vi "Log_ADAM_scan_table.vi"() -> ()   [LabVIEW 2012]
uses:
  ADAM Client/Sub VIs/ADAM Controls/Channel_State.ctl
  Anemometry/Anemometry Sub Vis/Globals/Constants_global.vi
  Anemometry/Anemometry Sub Vis/Globals/Preference_global.vi
  ADAM_Global.vi
  Anemometry/Anemometry Sub Vis/Globals/Meas_global.vi
panel:
  in  "Averaging time (Seconds)":dbl=60.0
  out "Current time":string
  out "Started Time":string
  in  "stop":bool
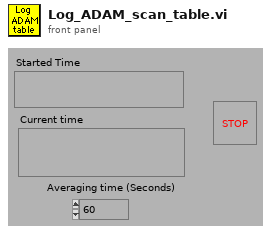
[diagram p1: front panel]
types:
  T1 = enum16{"On", "Off", "Always On", "Always Off", "Delete"}
  T2 = typedef "Channel_State.ctl" = enum16{"On", "Off", "Always On", "Always Off"}
  T3 = enum16{"Load ADAM setup from excel file", "Save ADAM setup to excel file"}
  T4 = cluster{"second":i32, "minute":i32, "hour":i32, "day of month":i32, "month":i32, "year":i32, "day of week":i32, "day of year":i32, "is DST":i32}
  T5 = typedef "Client_State_Cluster.ctl" = cluster{"Client Name":string, "Traverse level State":T6, "People to Email":string[], "Next Contact Time":dbl}
  T6 = typedef "Traverse_Level_State.ctl" = enum16{"Running", "Complete"}
  T7 = typedef "Server_Control.ctl" = cluster{"Channel Name to control":string, "Channel sharing":enum16{"Channel Unshared", "Channel Shared by Rig", "Channel Shared by Group"}, "Default Value":dbl, "Client Array":string[], "Time Stamp":timestamp, "Do Not Reset":bool}
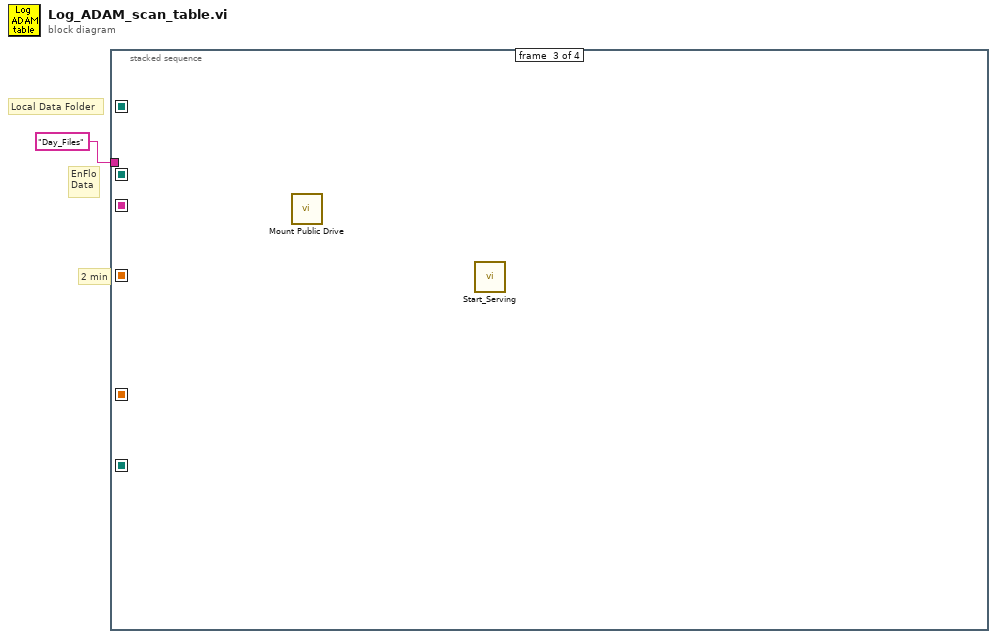
[diagram p0: block diagram]
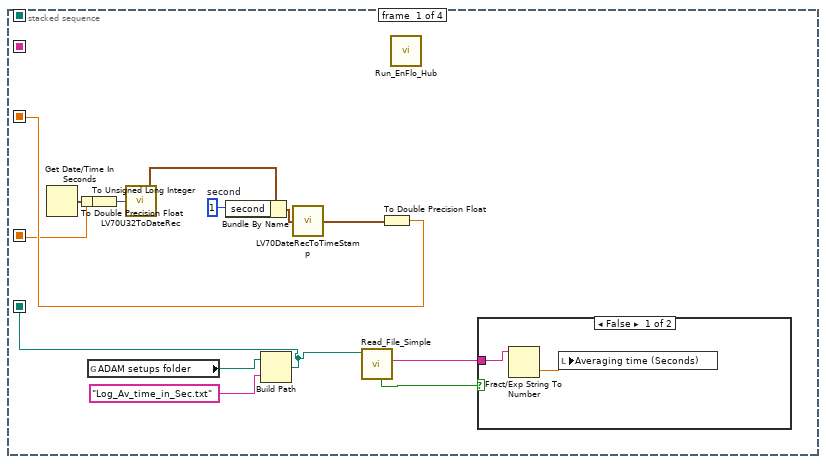
[diagram p2: hidden frame]
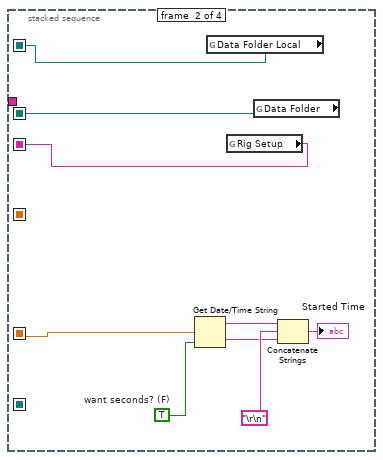
[diagram p4: hidden frame]
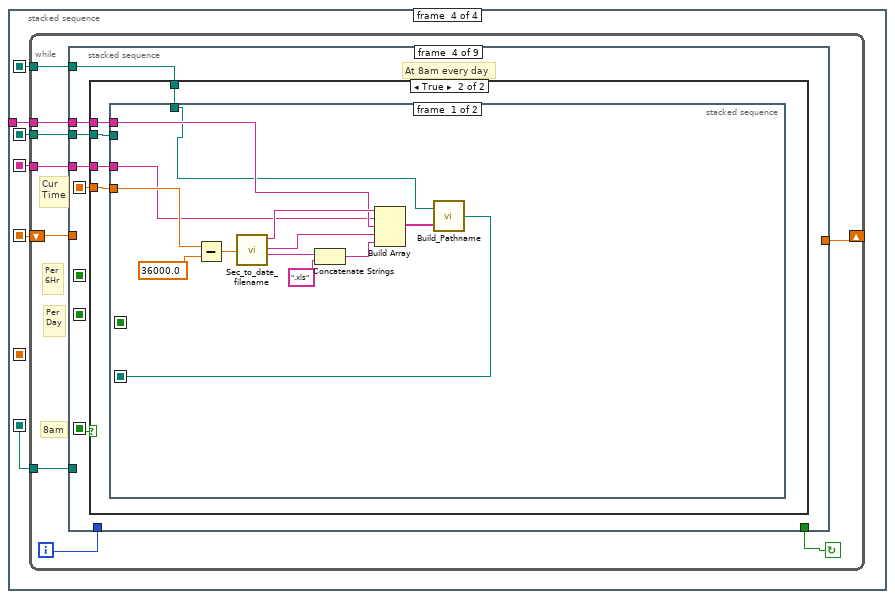
[diagram p5: hidden frame]
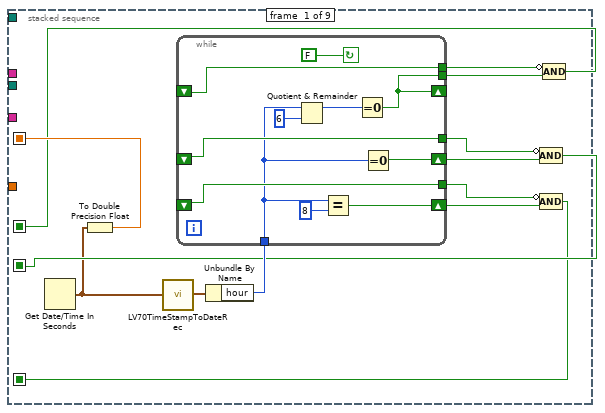
[diagram p6: hidden frame]
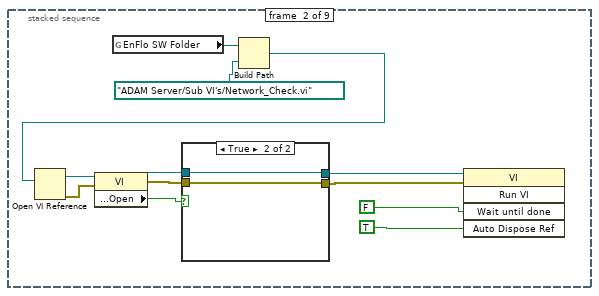
[diagram p7: hidden frame]
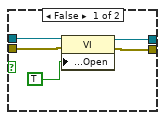
[diagram p8: hidden frame]
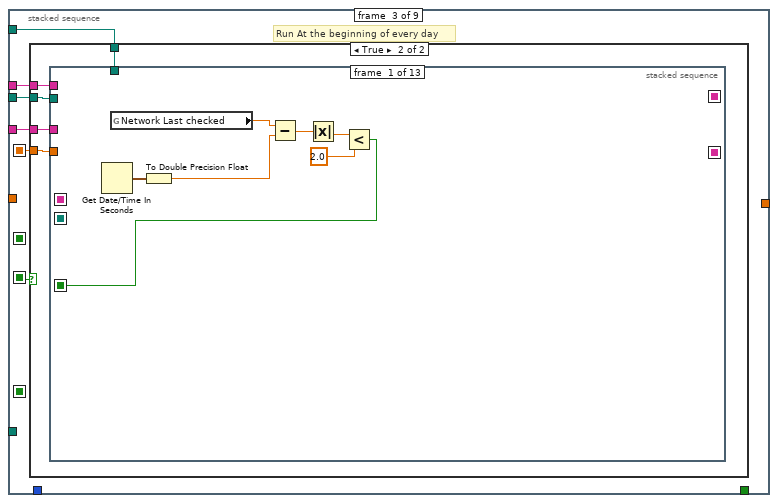
[diagram p9: hidden frame]
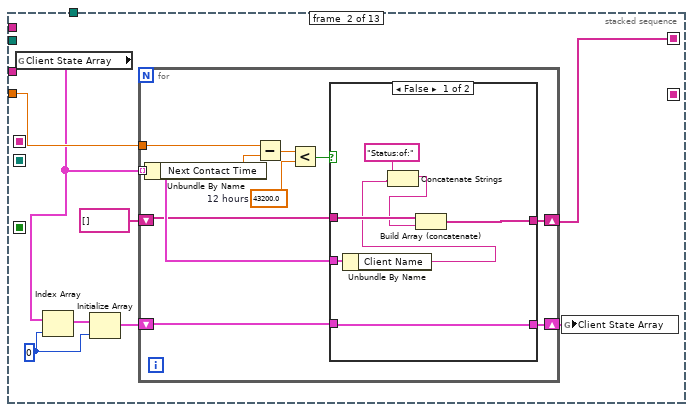
[diagram p11: hidden frame]
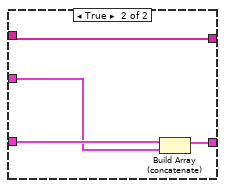
[diagram p12: hidden frame]
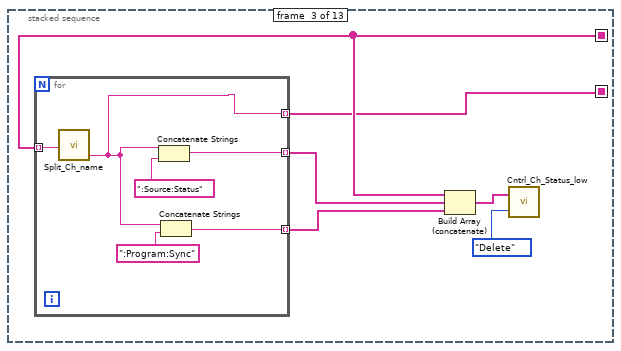
[diagram p13: hidden frame]
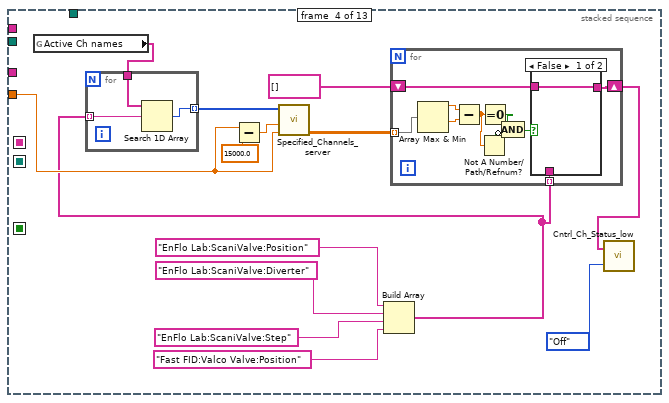
[diagram p14: hidden frame]
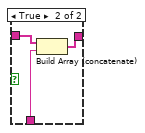
[diagram p15: hidden frame]
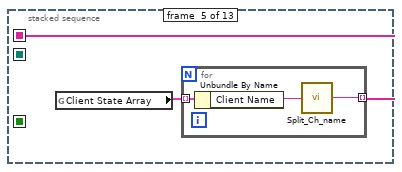
[diagram p16: hidden frame]
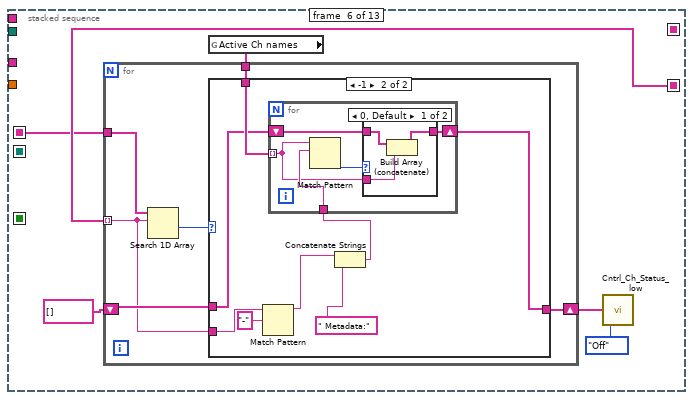
[diagram p17: hidden frame]
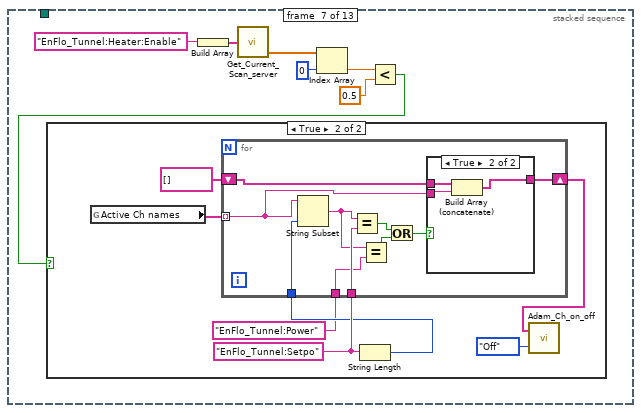
[diagram p20: hidden frame]
diagram:
  # "Local Data Folder"
  # "EnFlo\nData"
  # "2 min"
  n1 = stacked-sequence {
    seq-local: [w12 _ _ _] -> [_ _ _ w31]
    seq-local: [w11 _ _ _] -> [_ w25 _ _]
    seq-local: [_ w19 _ _] -> [_ _ _ w30]
    seq-local: [w4 _ _ _] -> [_ _ _ w28]
    seq-local: [_ w18 _ _] -> [_ _ _ w27]
    seq-local: [_ w17 _ _] -> [_ _ _ w26]
    tunnel: "Day_Files" ("Input Element") -> [_ _ _ w29]
    frame #0 {
      w14 = 1  # second
      n2 = Get Date/Time In Seconds() -> (seconds since 1Jan1904=w8:timestamp)
      n3 = To Double Precision Float(number=w8) -> (double precision float=w11:dbl)
      n4 = global read "Constants_global.vi" "ADAM setups folder"() -> (w6:path)
      n5 = To Unsigned Long Integer(number=w11) -> (unsigned 32bit integer=w10:u32)
      n6 = call <vilib>:"LV70U32ToDateRec.vi"("Time"=w10) -> ("date time rec"=w9:T4)
      n7 = Bundle By Name(cluster=w9, "second"=w14) -> (w13:T4)
      n8 = Build Path(base path=w6, name or relative path="Log_Av_time_in_Sec.txt") -> (appended path=w4:path)
      n9 = call <vilib>:"LV70DateRecToTimeStamp.vi"("date time rec"=w13) -> ("Time Stamp"=w7:timestamp)
      n10 = call "Read_File_Simple.vi"("Filename"=w4) -> ("Error?"=w2:bool, "string"=w3:string)  [unwired: 2 in, 6 out]
      n11 = To Double Precision Float(number=w7) -> (double precision float=w12:dbl)
      n12 = call "Run_EnFlo_Hub.vi"() -> ()  [unwired: 8 out]
      n13 = case shown="False" w2 {
        tunnel: w3 -> [w16 _]
        frame False {
          n14 = Fract/Exp String To Number(string=w16) -> (number=w15:dbl)  [unwired: 4 out]
          n15 = local write "Averaging time (Seconds)"(w15) -> ()
        }
        frame True {
        }
      }
    }
    frame #1 {
      w24 = TRUE  # want seconds? (F)
      n16 = Get Date/Time String(seconds (now)=w25, want seconds? (F)=w24) -> (date string=w22:string, time string=w21:string)  [unwired: 1 out]
      n17 = global read "Constants_global.vi" "Data Folder Local"() -> (w17:path)
      n18 = global read "Preference_global.vi" "Rig Setup"() -> (w18:string)
      n19 = global read "Constants_global.vi" "Data Folder"() -> (w19:path)
      n20 = Concatenate Strings(w22, "\r\n", w21) -> (→"Started Time":string)
    }
    frame #2 {
      n21 = call "Mount Public Drive.vi"() -> ()  [unwired: 12 in]
      n22 = call "Start_Serving.vi"() -> ()  [unwired: 1 out]
    }
    frame #3 {
      n23 = while {
        tunnel: w30 -> [w38]
        shift-left: w31 -> [w40]
        shift-right: [w39] -> _
        tunnel: w29 -> [w35]
        tunnel: w28 -> [w34]
        tunnel: w27 -> [w33]
        tunnel: w26 -> [w32]
        i -> [w37]
        stop <- w36 continue-if-true
        # "8am"
        # "Per\n6Hr"
        # "Per\nDay"
        # "Cur\nTime"
        n24 = stacked-sequence {
          seq-local: [w45 _ _ _ _ _ _ _ _] -> [_ _ w89 _ _ _ _ _ _]
          seq-local: [w52 _ _ _ _ _ _ _ _] -> [_ _ w88 w329 w366 w380 w384 _ _]
          seq-local: [w48 _ _ _ _ _ _ _ _] -> [_ _ _ _ w360 _ _ _ _]
          seq-local: [w41 _ _ _ _ _ _ _ _] -> [_ _ _ w324 _ _ _ _ _]
          tunnel: [_ _ _ _ _ _ w383 _ _] -> w39
          tunnel: w40 -> [_ _ _ _ _ _ w385 _ _]
          tunnel: w38 -> [_ _ w87 w328 _ _ w392 _ _]
          tunnel: w37 -> [_ _ _ _ w359 _ _ _ _]
          tunnel: [_ _ _ _ _ _ _ _ w441] -> w36
          tunnel: w35 -> [_ _ w86 w327 _ _ w393 _ _]
          tunnel: w34 -> [_ _ _ _ _ _ _ _ w440]
          tunnel: w33 -> [_ _ w85 w326 _ _ w386 _ _]
          tunnel: w32 -> [_ _ w84 w325 _ _ w382 _ _]
          frame #0 {
            n25 = Get Date/Time In Seconds() -> (seconds since 1Jan1904=w44:timestamp)
            n26 = To Double Precision Float(number=w44) -> (double precision float=w52:dbl)
            n27 = call <vilib>:"LV70TimeStampToDateRec.vi"("time stamp"=w44) -> ("date time rec"=w53:T4)
            n28 = Unbundle By Name(w53) -> ("hour"=w51:i32)
            n29 = while {
              tunnel: [w59] -> w46
              shift-left: _ -> [w59]
              shift-right: [w60] -> w47
              tunnel: [w61] -> w49
              tunnel: [w62] -> w50
              tunnel: w51 -> [w56]
              shift-left: _ -> [w61]
              shift-right: [w62] -> _
              tunnel: [w57] -> w43
              shift-right: [w54] -> w42
              shift-left: _ -> [w57]
              stop <- FALSE continue-if-true
              n30 = Quotient & Remainder(x=w56, y=6) -> (x-y*floor(x/y)=w63:i32)  [unwired: 1 out]
              n31 = Equal?(x=w56, y=8) -> (x = y?=w54:bool)
              n32 = Equal To 0?(x=w63) -> (x = 0?=w62:bool)
              n33 = Equal To 0?(x=w56) -> (x = 0?=w60:bool)
            }
            n34 = Compound Arithmetic op=AND(invert w46, w47) -> (w45:bool)
            n35 = Compound Arithmetic op=AND(invert w43, w42) -> (w41:bool)
            n36 = Compound Arithmetic op=AND(invert w49, w50) -> (w48:bool)
          }
          frame #1 {
            n37 = global read "Constants_global.vi" "EnFlo SW Folder"() -> (w74:path)
            n38 = Build Path(base path=w74, name or relative path=path "ADAM Server/Sub VI's/Network_Check.vi") -> (appended path=w75:path)
            n39 = Open VI Reference(vi path=w75) -> (vi reference=w71:refnum<vi>, error out=w70:errorcluster)  [unwired: 1 in, 4 out]
            n40 = property class="VI"(reference=w71, error in=w70) -> (reference out=w68:refnum<vi>, error out=w67:errorcluster, "Front Panel Window:Open"=w69:bool)
            n41 = case shown="True" w69 {
              tunnel: w68 -> [w80 w83]
              tunnel: w67 -> [w79 w82]
              tunnel: [w78 w83] -> w66
              tunnel: [w77 w82] -> w65
              frame False {
                n42 = property class="VI"(reference=w80, error in=w79, "Front Panel Window:Open"=TRUE) -> (reference out=w78:refnum<vi>, error out=w77:errorcluster)
              }
              frame True {
              }
            }
            n43 = invoke class="VI" method="Run VI"(reference=w66, error in=w65, "Wait until done"=FALSE, "Auto Dispose Ref"=TRUE) -> ()  [unwired: 1 in, 5 out]
          }
          frame #2 {
            # "Run At the beginning of every day"
            n44 = case shown="True" w89 {
              tunnel: w88 -> [_ w94]
              tunnel: w87 -> [_ w93]
              tunnel: w86 -> [_ w92]
              tunnel: w85 -> [_ w91]
              tunnel: w84 -> [_ w90]
              frame False {
              }
              frame True {
                n45 = stacked-sequence {
                  seq-local: [_ w102 _ _ _ _ _ _ _ _ _ _ _] -> [_ _ w136 _ _ _ _ _ _ w257 _ _ _]
                  seq-local: [_ _ w132 _ _ _ _ _ _ _ _ _ _] -> [_ _ _ _ _ w184 _ _ _ _ _ _ _]
                  seq-local: [_ _ _ _ w174 _ _ _ _ _ _ _ _] -> [_ _ _ _ _ w181 _ _ _ _ _ _ _]
                  seq-local: [_ _ _ _ _ _ _ _ _ _ _ w307 _] -> [_ _ _ _ _ _ _ _ _ _ _ _ w310]
                  seq-local: [w95 _ _ _ _ _ _ _ _ _ _ _ _] -> [_ _ _ _ _ _ _ w237 _ _ w285 _ w309]
                  tunnel: w94 -> [_ w109 _ w153 _ _ _ _ _ _ w286 _ w311]
                  tunnel: w93 -> [_ _ _ _ _ _ _ _ _ _ _ _ _]
                  tunnel: w92 -> [_ _ _ _ _ _ _ _ _ _ _ _ _]
                  tunnel: w91 -> [_ _ _ _ _ _ _ _ _ _ _ _ _]
                  tunnel: w90 -> [_ _ _ _ _ _ _ _ _ _ _ _ _]
                  frame #0 {
                    n46 = Get Date/Time In Seconds() -> (seconds since 1Jan1904=w100:timestamp)
                    n47 = global read "ADAM_Global.vi" "Network Last checked"() -> (w97:dbl)
                    n48 = To Double Precision Float(number=w100) -> (double precision float=w101:dbl)
                    n49 = Subtract(x=w97, y=w101) -> (x-y=w98:dbl)
                    n50 = Absolute Value(x=w98) -> (abs(x)=w96:dbl)
                    n51 = Less?(x=w96, y=2.0) -> (x < y?=w95:bool)
                  }
                  frame #1 {
                    w107 = 0 ("Index")
                    n52 = global read "ADAM_Global.vi" "Client State Array"() -> (w108:T5[])
                    n53 = Index Array(array=w108, index=w107) -> (element=w106:T5)
                    n54 = Initialize Array(w106, w107) -> (w105:T5[])
                    n55 = for {
                      tunnel: w108 -> [w112] mode=indexing
                      shift-right: [w113] -> w104
                      shift-left: w105 -> [w114]
                      tunnel: w109 -> [w119]
                      shift-right: [w110] -> w102
                      shift-left: string[] [] -> [w111]
                      w116 = 43200.0  # 12 hours
                      n56 = Unbundle By Name(w112) -> ("Next Contact Time"=w118:dbl)
                      n57 = Subtract(x=w119, y=w118) -> (x-y=w117:dbl)
                      n58 = Less?(x=w117, y=w116) -> (x < y?=w115:bool)
                      n59 = case shown="False" w115 {
                        tunnel: w114 -> [w126 w130]
                        tunnel: [w126 w129] -> w113
                        tunnel: w112 -> [w125 w128]
                        tunnel: w111 -> [w124 w127]
                        tunnel: [w123 w127] -> w110
                        frame False {
                          n60 = Unbundle By Name(w125) -> ("Client Name"=w121:string)
                          n61 = Concatenate Strings("Status:of:", w121) -> (w120:string)
                          n62 = Build Array (concatenate)(w124, w120) -> (w123:string[])
                        }
                        frame True {
                          n63 = Build Array (concatenate)(w130, w128) -> (w129:T5[])
                        }
                      }
                    }
                    n64 = global write "ADAM_Global.vi" "Client State Array"(w104) -> ()
                  }
                  frame #2 {
                    n65 = for {
                      tunnel: w136 -> [w142] mode=indexing
                      tunnel: [w139] -> w134 mode=indexing
                      tunnel: [w138] -> w133 mode=indexing
                      tunnel: [w137] -> w132 mode=indexing
                      n66 = call "Split_Ch_name.vi"("Ch name"=w142) -> ("Low level"=w137:string)  [unwired: 2 out]
                      n67 = Concatenate Strings(w137, ":Source:Status") -> (w139:string)
                      n68 = Concatenate Strings(w137, ":Program:Sync") -> (w138:string)
                    }
                    n69 = Build Array (concatenate)(w136, w134, w133) -> (w135:string[])
                    n70 = call "Cntrl_Ch_Status_low.vi"("Mode"=T1."Delete", "Channel names"=w135) -> ()  [unwired: 1 out]
                  }
                  frame #3 {
                    n71 = global read "ADAM_Global.vi" "Active Ch names"() -> (w156:string[])
                    n72 = Subtract(x=w153, y=15000.0) -> (x-y=w151:dbl)
                    n73 = Build Array("EnFlo Lab:ScaniValve:Position", "EnFlo Lab:ScaniValve:Diverter", "EnFlo Lab:ScaniValve:Step", "Fast FID:Valco Valve:Position") -> (w149:string[])
                    n74 = for {
                      tunnel: w156 -> [w173]
                      tunnel: w149 -> [w172] mode=indexing
                      tunnel: [w171] -> w154 mode=indexing
                      n75 = Search 1D Array(1D array=w173, element=w172) -> (index of element=w171:i32)  [unwired: 1 out]
                    }
                    n76 = call "Specified_Channels_server.vi"("End time"=w153, "Start time"=w151, "Requested channels"=w154) -> ("Output array"=w150:dbl[][])  [unwired: 2 in, 4 out]
                    n77 = for {
                      tunnel: w150 -> [w163] mode=indexing
                      shift-right: [w164] -> w144
                      shift-left: string[] [] -> [w158]
                      tunnel: w149 -> [w159] mode=indexing
                      n78 = Array Max & Min(array=w163) -> (max value=w166:dbl, min value=w165:dbl)  [unwired: 2 out]
                      n79 = Subtract(x=w166, y=w165) -> (x-y=w162:dbl)
                      n80 = Not A Number/Path/Refnum?(number/path/refnum=w162) -> (NaN/Path/Refnum?=w160:bool)
                      n81 = Equal To 0?(x=w162) -> (x = 0?=w157:bool)
                      n82 = Compound Arithmetic op=AND(w157, invert w160) -> (w161:bool)
                      n83 = case shown="False" w161 {
                        tunnel: [w167 w170] -> w164
                        tunnel: w159 -> [_ w169]
                        tunnel: w158 -> [w167 w168]
                        frame False {
                        }
                        frame True {
                          n84 = Build Array (concatenate)(w168, w169) -> (w170:string[])
                        }
                      }
                    }
                    n85 = call "Cntrl_Ch_Status_low.vi"("Mode"=T1."Off", "Channel names"=w144) -> ()  [unwired: 1 out]
                  }
                  frame #4 {
                    n86 = global read "ADAM_Global.vi" "Client State Array"() -> (w175:T5[])
                    n87 = for {
                      tunnel: w175 -> [w178] mode=indexing
                      tunnel: [w176] -> w174 mode=indexing
                      n88 = Unbundle By Name(w178) -> ("Client Name"=w177:string)
                      n89 = call "Split_Ch_name.vi"("Ch name"=w177) -> ("Middle"=w176:string)  [unwired: 2 out]
                    }
                  }
                  frame #5 {
                    n90 = global read "ADAM_Global.vi" "Active Ch names"() -> (w182:string[])
                    n91 = for {
                      tunnel: w184 -> [w185] mode=indexing
                      shift-right: [w188] -> w180
                      shift-left: string[] [] -> [w189]
                      tunnel: w182 -> [w187]
                      tunnel: w181 -> [w186]
                      n92 = Search 1D Array(1D array=w186, element=w185) -> (index of element=w190:i32)  [unwired: 1 out]
                      n93 = case shown="-1" w190 {
                        tunnel: w189 -> [w191 w197]
                        tunnel: [w191 w196] -> w188
                        tunnel: w185 -> [_ w192]
                        tunnel: w187 -> [_ w198]
                        frame 0, Default {
                        }
                        frame -1 {
                          n94 = Match Pattern(string=w192, regular expression="-") -> (before substring=w193:string)  [unwired: 4 out]
                          n95 = Concatenate Strings(w193, " Metadata:" ("Substring")) -> (w195:string)
                          n96 = for {
                            shift-right: [w202] -> w196
                            shift-left: w197 -> [w203]
                            tunnel: w195 -> [w201]
                            tunnel: w198 -> [w200] mode=indexing
                            n97 = Match Pattern(string=w200, regular expression=w201) -> (offset past match=w204:i32)  [unwired: 4 out]
                            n98 = case shown="0, Default" w204 {
                              tunnel: w203 -> [w206 w208]
                              tunnel: [w205 w208] -> w202
                              tunnel: w200 -> [w207 _]
                              frame 0, Default {
                                n99 = Build Array (concatenate)(w206, w207) -> (w205:string[])
                              }
                              frame -1 {
                              }
                            }
                          }
                        }
                      }
                    }
                    n100 = call "Cntrl_Ch_Status_low.vi"("Mode"=T1."Off", "Channel names"=w180) -> ()  [unwired: 1 out]
                  }
                  frame #6 {
                    n101 = Build Array("EnFlo_Tunnel:Heater:Enable") -> (w214:string[])
                    n102 = call "Get_Current_Scan_server.vi"("Desired Channels"=w214) -> ("Numerical Values"=w213:dbl[])  [unwired: 2 out]
                    n103 = Index Array(array=w213, index=0) -> (element=w211:dbl)
                    n104 = Less?(x=w211, y=0.5) -> (x < y?=w209:bool)
                    n105 = case shown="True" w209 {
                      frame False {
                      }
                      frame True {
                        w220 = "EnFlo_Tunnel:Setpo"
                        n106 = global read "ADAM_Global.vi" "Active Ch names"() -> (w218:string[])
                        n107 = String Length(string=w220) -> (length=w219:i32)
                        n108 = for {
                          shift-right: [w228] -> w217
                          shift-left: string[] [] -> [w230]
                          tunnel: w218 -> [w229] mode=indexing
                          tunnel: w219 -> [w232]
                          tunnel: w220 -> [w231]
                          tunnel: "EnFlo_Tunnel:Power" -> [w226]
                          n109 = String Subset(string=w229, length (rest)=w232) -> (substring=w227:string)  [unwired: 1 out]
                          n110 = Equal?(x=w227, y=w231) -> (x = y?=w224:bool)
                          n111 = Equal?(x=w227, y=w226) -> (x = y?=w225:bool)
                          n112 = Or(x=w224, y=w225) -> (x .or. y?=w223:bool)
                          n113 = case shown="True" w223 {
                            tunnel: w230 -> [w233 w236]
                            tunnel: w229 -> [_ w235]
                            tunnel: [w233 w234] -> w228
                            frame False {
                            }
                            frame True {
                              n114 = Build Array (concatenate)(w236, w235) -> (w234:string[])
                            }
                          }
                        }
                        n115 = call "Adam_Ch_on_off.vi"("Ch State"=Channel_State."Off", "ADAM Ch Names"=w217) -> ()  [unwired: 1 out]
                      }
                    }
                  }
                  frame #7 {
                    n116 = case shown="True" w237 {
                      frame False {
                      }
                      frame True {
                        n117 = call "Read_Write_ADAM_setup.vi"("Mode"=T3."Save ADAM setup to excel file") -> ()  [unwired: 4 out]
                      }
                    }
                  }
                  frame #8 {
                    w242 = 5400.0  # 1.5 Hrs in seconds
                    n118 = Build Array("GMU:Source:Meas Q", "GMU:Source:Est Time") -> (w249:string[])
                    n119 = call "Get_Current_Scan_server.vi"("Desired Channels"=w249) -> ("Numerical Values"=w244:dbl[])  [unwired: 2 out]
                    n120 = Index Array(array=w244, index=0 ("Index")) -> (element=w246:dbl)
                    n121 = Index Array(array=w244, index=1 ("Index")) -> (element=w243:dbl)
                    n122 = Less?(x=w246, y=0.01) -> (x < y?=w240:bool)
                    n123 = Greater?(x=w243, y=w242) -> (0:w241:bool)
                    n124 = And(x=w240, y=w241) -> (x .and. y?=w239:bool)
                    n125 = case shown="True" w239 {
                      frame False {
                      }
                      frame True {
                        w252 = FALSE  # Activate channels
                        w253 = enum16{"Channel Name", "Main Address"}."Channel Name" ("Control on")
                        n126 = call "Ch_Active_Control.vi"("Match"="GMU:", "Activate Channels?"=w252, "Control on"=w253) -> ()  [unwired: 1 in, 2 out]
                        n127 = call "Ch_Active_Control.vi"("Match"="source", "Activate Channels?"=w252, "Control on"=w253) -> ()  [unwired: 1 in, 2 out]
                      }
                    }
                  }
                  frame #9 {
                    w261 = 0 ("Index")
                    n128 = global read "ADAM_Global.vi" "Server Control Array"() -> (w258:T7[])
                    n129 = Index Array(array=w258, index=w261) -> (element=w260:T7)
                    n130 = Initialize Array(w260, w261) -> (w259:T7[])
                    n131 = for {
                      tunnel: w258 -> [w263] mode=indexing
                      shift-right: [w268] -> w256
                      shift-left: w259 -> [w269]
                      tunnel: w257 -> [w267]
                      n132 = Unbundle By Name(w263) -> ("Client Array"=w266:string[])
                      n133 = for {
                        tunnel: w267 -> [w274]
                        tunnel: w266 -> [w272] mode=indexing
                        shift-right: [w270] -> w262
                        shift-left: string[] [] -> [w271]
                        n134 = Search 1D Array(1D array=w274, element=w272) -> (index of element=w273:i32)  [unwired: 1 out]
                        n135 = case shown="0, Default" w273 {
                          tunnel: w272 -> [_ w278]
                          tunnel: w271 -> [w275 w277]
                          tunnel: [w275 w276] -> w270
                          frame 0, Default {
                          }
                          frame -1 {
                            n136 = Build Array (concatenate)(w277, w278) -> (w276:string[])
                          }
                        }
                      }
                      n137 = Array Size(array=w262) -> (size(s)=w264:i32)
                      n138 = case shown="0" w264 {
                        tunnel: w269 -> [w279 w283]
                        tunnel: [w279 w284] -> w268
                        tunnel: w263 -> [_ w282]
                        tunnel: w262 -> [_ w281]
                        frame 0 {
                        }
                        frame 1, Default {
                          n139 = Bundle By Name(cluster=w282, "Client Array"=w281) -> (w280:T7)
                          n140 = Build Array (concatenate)(w283, w280) -> (w284:T7[])
                        }
                      }
                    }
                    n141 = global write "ADAM_Global.vi" "Server Control Array"(w256) -> ()
                  }
                  frame #10 {
                    n142 = case shown="True" w285 {
                      frame False {
                      }
                      frame True {
                        w294 = "\r\n"
                        n143 = global read "Constants_global.vi" "ADAM setups folder"() -> (w297:path)
                        n144 = Build Path(base path=w297, name or relative path="Setup_Files") -> (appended path=w301:path)
                        n145 = Build Path(base path=w297, name or relative path="Hi_Tec_Calibs.xls") -> (appended path=w296:path)
                        n146 = Build Path(base path=w301, name or relative path="Selected_Filename.txt" ("Substring")) -> (appended path=w303:path)
                        n147 = call "Read_File_Simple.vi"("Filename"=w303) -> ("string"=w302:string)  [unwired: 2 in, 7 out]
                        n148 = Build Path(base path=w301, name or relative path=w302) -> (appended path=w300:path)
                        n149 = call "Read_File_Simple.vi"("Filename"=w296) -> ("string"=w295:string)  [unwired: 2 in, 7 out]
                        n150 = call "Read_File_Simple.vi"("Filename"=w300) -> ("string"=w299:string)  [unwired: 2 in, 7 out]
                        n151 = call "Get_mod_dates.vi"() -> ("Output string"=w293:string)  [unwired: 1 in, 4 out]
                        n152 = call "Create_Error_log_folders.vi"("Per Day Log File?"=TRUE, "Log Filename"="ADAM_Setups" ("Substring")) -> ("Server copy Location"=w287:path, "Local Log File"=w289:path)  [unwired: 1 in, 1 out]
                        n153 = Concatenate Strings(w299, w294, w295, w294, w293) -> (w290:string)
                        n154 = call "Write_File_Simple.vi"("character string"=w290, "file path"=w289) -> ("file path Out"=w288:path)  [unwired: 1 in, 1 out]
                        n155 = call "Updated_File_Copy.vi"("Target Path"=w287, "Source Path"=w288) -> ()  [unwired: 2 out]
                      }
                    }
                    n156 = global write "Meas_global.vi" "Start Time of experiment"(w286) -> ()
                  }
                  frame #11 {
                    n157 = global read "Constants_global.vi" "Data Folder Local"() -> (w308:path)
                    n158 = Build Path(base path=w308, name or relative path="Results_Summary_files") -> (appended path=w307:path)
                  }
                  frame #12 {
                    n159 = case shown="True" w309 {
                      tunnel: w311 -> [_ w314]
                      tunnel: w310 -> [_ w312]
                      frame False {
                      }
                      frame True {
                        # "If the summary files are more than 60 days old delete them"
                        n160 = To Unsigned Long Integer(number=w314) -> (unsigned 32bit integer=w313:u32)
                        n161 = call "Get_folder_and_filenames.vi"("file path (dialog if empty)"=w312) -> ("Files"=w315:path[])  [unwired: 1 out]
                        n162 = for {
                          tunnel: w315 -> [w317] mode=indexing
                          tunnel: w313 -> [w322]
                          # "60 days in seconds"
                          n163 = File/Directory Info(path=w317) -> (last mod=w316:timestamp)  [unwired: 1 in, 6 out]
                          n164 = To Unsigned Long Integer(number=w316) -> (unsigned 32bit integer=w321:u32)
                          n165 = Subtract(x=w322, y=w321) -> (x-y=w320:u32)
                          n166 = Greater?(x=w320, y=u32 5184000) -> (0:w318:bool)
                          n167 = case shown="False" w318 {
                            tunnel: w317 -> [_ w323]
                            frame False {
                            }
                            frame True {
                              n168 = Delete(path (use dialog)=w323) -> ()  [unwired: 1 in, 6 out]
                            }
                          }
                        }
                      }
                    }
                  }
                }
              }
            }
          }
          frame #3 {
            # "At 8am every day"
            n169 = case shown="True" w324 {
              tunnel: w329 -> [_ w334]
              tunnel: w328 -> [_ w333]
              tunnel: w327 -> [_ w332]
              tunnel: w326 -> [_ w331]
              tunnel: w325 -> [_ w330]
              frame False {
              }
              frame True {
                n170 = stacked-sequence {
                  seq-local: [w342 _] -> [_ w355]
                  seq-local: [_ w348] -> [_ _]
                  tunnel: w334 -> [w346 _]
                  tunnel: w333 -> [_ _]
                  tunnel: w332 -> [w340 _]
                  tunnel: w331 -> [w336 _]
                  tunnel: w330 -> [w335 _]
                  frame #0 {
                    n171 = Subtract(x=w346, y=36000.0) -> (x-y=w344:dbl)
                    n172 = call "Sec_to_date_filename.vi"("seconds"=w344) -> ("Year"=w341:string, "Month"=w345:string, "Day"=w338:string)  [unwired: 1 out]
                    n173 = Concatenate Strings(w338, ".xls" ("string")) -> (w337:string)
                    n174 = Build Array(w341, w336, w340, w345, w337) -> (w343:string[])
                    n175 = call "Build_Pathname.vi"("PathElements"=w343, "PathnameIn"=w335) -> ("AppendedPath"=w342:path)
                  }
                  frame #1 {
                    n176 = Get Date/Time In Seconds() -> (seconds since 1Jan1904=w353:timestamp)
                    n177 = global read "ADAM_Global.vi" "Network Last checked"() -> (w350:dbl)
                    n178 = To Double Precision Float(number=w353) -> (double precision float=w354:dbl)
                    n179 = Subtract(x=w350, y=w354) -> (x-y=w351:dbl)
                    n180 = Absolute Value(x=w351) -> (abs(x)=w349:dbl)
                    n181 = Less?(x=w349, y=2.0) -> (x < y?=w348:bool)
                    n182 = case shown="True" w348 {
                      tunnel: w355 -> [_ w356]
                      frame False {
                      }
                      frame True {
                        # "This VI emails a summary of all the server errors that occured Yesterday"
                        n183 = call "Adam_server_messages.vi"("Filename"=w356) -> ()  [unwired: 1 out]
                      }
                    }
                  }
                }
              }
            }
          }
          frame #4 {
            n184 = global read "ADAM_Global.vi" "Network Last checked"() -> (w365:dbl)
            n185 = Subtract(x=w366, y=w365) -> (x-y=w361:dbl)
            n186 = Greater?(x=w359, y=30) -> (0:w357:bool)
            n187 = Greater?(x=w361, y=25.0) -> (0:w363:bool)
            n188 = Compound Arithmetic op=AND(w363, w360, w357) -> (w362:bool)
            n189 = case shown="True" w362 {
              tunnel: w361 -> [_ w371]
              tunnel: w360 -> [w367 _]
              frame False {
                n190 = case shown="True" w367 {
                  frame False {
                  }
                  frame True {
                    n191 = call "Organise_Movies.vi"() -> ()  [unwired: 1 out]
                  }
                }
              }
              frame True {
                n192 = Divide(x=w371, y=60.0) -> (x/y=w369:dbl)
                n193 = global read "Constants_global.vi" "ADAM setups folder"() -> (w379:path)
                n194 = Path to Array of Strings(0:w379) -> (2:w373:string[])  [unwired: 1 out]
                n195 = Index Array(array=w373, index=0) -> (element=w375:string)
                n196 = Format Into String(format string="%s Offline", w375) -> (resulting string=w377:string)  [unwired: 2 in, 1 out]
                n197 = Format Into String(format string="The file %s has been Offline now for %d minutes", w379, w369) -> (resulting string=w368:string)  [unwired: 2 in, 1 out]
                n198 = call "Server_Emails.vi"("Message"=w368, "Contact All clients?"=TRUE, "Subject"=w377) -> ()  [unwired: 2 in, 3 out]
              }
            }
          }
          frame #5 {
            n199 = call "EnFlo_Seeder_Control.vi"("Current Time (s)"=w380) -> ()
            n200 = Wait (ms)(milliseconds to wait=u32 1000 ("milliseconds to Wait")) -> ()  [unwired: 1 out]
          }
          frame #6 {
            n201 = Divide(x="Averaging time (Seconds)", y=60.0) -> (x/y=w390:dbl)
            n202 = Divide(x="Averaging time (Seconds)", y=2.0) -> (x/y=w387:dbl)
            n203 = Add(x=w387, y=w385) -> (x+y=w403:dbl)
            n204 = call "Sec_to_date_filename.vi"("seconds"=w403) -> ("Year"=w398:string, "Month"=w399:string, "Day"=w394:string)  [unwired: 1 out]
            n205 = Concatenate Strings(w394, ".xls" ("string")) -> (w396:string)
            n206 = Build Array(w398, w386, w393, w399, w396) -> (w397:string[])
            n207 = call "Time_elapsed.vi"("End of previous average in"=w385, "Averaging time (mins)"=w390) -> ("End of previous average out"=w383:dbl, "End of period"=w401:dbl, "Start of period"=w402:dbl, "Time elapsed ?"=w400:bool)  [unwired: 2 in]
            n208 = case shown="True" w400 {
              tunnel: w401 -> [_ w408]
              tunnel: w402 -> [_ w409]
              tunnel: w392 -> [_ w407]
              tunnel: w397 -> [_ w406]
              tunnel: w382 -> [_ w405]
              tunnel: w384 -> [_ w404]
              frame False {
              }
              frame True {
                n209 = stacked-sequence {
                  seq-local: [w410 _ _] -> [_ _ w429]
                  seq-local: [w412 _ _] -> [_ _ w431]
                  tunnel: w409 -> [w426 _ _]
                  tunnel: w408 -> [w425 _ _]
                  tunnel: w407 -> [_ _ w430]
                  tunnel: w406 -> [w421 _ w432]
                  tunnel: w405 -> [w420 _ _]
                  tunnel: w404 -> [w418 _ _]
                  frame #0 {
                    n210 = global read "ADAM_Global.vi" "Network Last checked"() -> (w419:dbl)
                    n211 = global read "ADAM_Global.vi" "2 Min average comment"() -> (w424:string)
                    n212 = global read "Meas_global.vi" "Error Messages"() -> (w423:string)
                    n213 = call "Build_Pathname.vi"("PathElements"=w421, "PathnameIn"=w420) -> ("AppendedPath"=w411:path)
                    n214 = call "Create_directory_path.vi"("Path name"=w411) -> ("Path name Out"=w410:path)  [unwired: 1 in, 1 out]
                    n215 = Subtract(x=w419, y=w418) -> (x-y=w417:dbl)
                    n216 = Concatenate Strings(w424, w423) -> (w422:string)
                    n217 = call "Write_to_log_file.vi"("User added comment"=w422, "End time"=w425, "Start time"=w426, "Folder/file"=w410) -> ("File Updated?"=w414:bool)  [unwired: 5 in, 2 out]
                    n218 = Absolute Value(x=w417) -> (abs(x)=w416:dbl)
                    n219 = Less?(x=w416, y=1.5) -> (x < y?=w413:bool)
                    n220 = And(x=w414, y=w413) -> (x .and. y?=w412:bool)
                  }
                  frame #1 {
                    w427 = ""
                    n221 = global write "ADAM_Global.vi" "2 Min average comment"(w427) -> ()
                    n222 = global write "Meas_global.vi" "Error Messages"(w427) -> ()
                  }
                  frame #2 {
                    n223 = call "Build_Pathname.vi"("PathElements"=w432, "PathnameIn"=w430) -> ("AppendedPath"=w428:path)
                    n224 = case shown="True" w431 {
                      tunnel: w429 -> [_ w434]
                      tunnel: w428 -> [_ w433]
                      frame False {
                      }
                      frame True {
                        n225 = call "Updated_File_Copy.vi"("Target Path"=w433, "Source Path"=w434) -> ()  [unwired: 2 out]
                      }
                    }
                  }
                }
              }
            }
          }
          frame #7 {
            w439 = TRUE  # want seconds? (F)
            n226 = Get Date/Time String(want seconds? (F)=w439) -> (date string=w437:string, time string=w436:string)  [unwired: 2 out]
            n227 = Concatenate Strings(w437, "\r\n", w436) -> (→"Current time":string)
          }
          frame #8 {
            n228 = while {
              shift-right: [w443] -> _
              shift-left: _ -> [w447]
              tunnel: w440 -> [w444]
              stop <- TRUE stop-if-true
              n229 = local read "Averaging time (Seconds)"() -> (w443:dbl)
              n230 = Not Equal?(x=w443, y=w447) -> (x != y?=w445:bool)
              n231 = case shown="True" w445 {
                tunnel: w444 -> [_ w448]
                tunnel: w443 -> [_ w450]
                frame False {
                }
                frame True {
                  n232 = Number To Fractional String(number=w450, precision (6)=i16 6) -> (F-format string=w449:string)  [unwired: 2 out]
                  n233 = call "Write_File_Simple.vi"("character string"=w449, "file path"=w448) -> ()  [unwired: 1 in, 2 out]
                }
              }
            }
            n234 = Not(x="stop") -> (.not. x?=w441:bool)
          }
        }
      }
    }
  }
